vi "Register with Manager.vi"(8 "error in (no error)":errorcluster, 11 "HistorianCharting in":refnum<class "HistorianCharting.lvclass">) -> (0 "error out":errorcluster, 2 "Group Events":refnum<event-registration>, 3 "HistorianCharting out":refnum<class "HistorianCharting.lvclass">)   [LabVIEW 2020, in "VolatusGUIElements.lvlib" / "HistorianCharting.lvclass"]
uses:
  HistorianCharting.lvclass
  VolatusGUI/Historian Charting Manager/Plot Group Events.ctl
  VolatusGUI/Historian Charting Manager/Plot Group Changed Data.ctl
  VolatusGUI/Historian Charting Manager/Plot Group Config.ctl
  VolatusGUI/Historian Charting Manager/X-Axis Type.ctl
  VolatusGUI/Historian Charting Manager/Plot Config.ctl
  VolatusGUI/Historian Charting Manager/Scale.ctl
  VolatusGUI/Historian Charting Manager/Plot Group Removed Data.ctl
  VolatusGUI/Historian Charting Manager/New Plot Group Data.ctl
  VolatusGUI/Historian Charting Manager/Chart Select Group Data.ctl
  VolatusGUI/Historian Charting Manager/Chart Registration.ctl
  VolatusGUI/Historian Charting Manager/Select Plot Group Data.ctl
  VolatusGUI/Plot Group Events Value/Plot Group Events Value.lvclass
  HistorianCharting.lvclass/HistorianCharting.ctl
  VolatusGUI/Plot Group Events Value/Plot Group Events Value.lvclass/Plot Group Events Value.ctl
  VolatusGUI/Historian Charting Manager/Historian Charting Manager.lvclass
  Volatus/MessageQ/MessageQ.lvclass
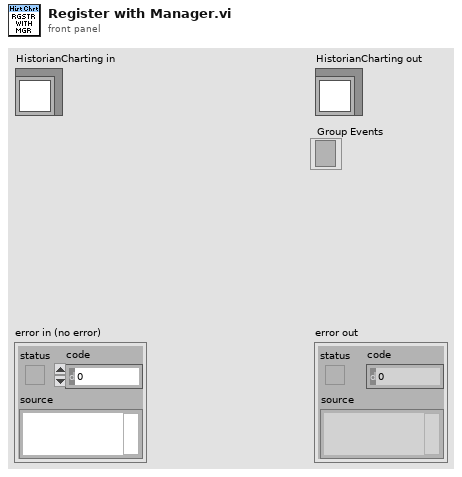
[diagram p1: front panel]
types:
  T1 = typedef "VolatusGUI.lvlib/Historian Charting Manager.lvclass/Chart Registration.ctl" = cluster{"Chart Num":i32, "Select Plot Group":refnum<user-event>}
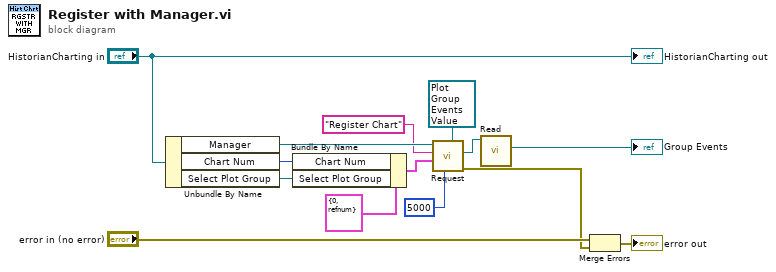
[diagram p0: block diagram]
diagram:
  n1 = Unbundle By Name("HistorianCharting in") -> ("Manager"=w9:refnum<class "MessageQ.lvclass">, "Chart Num"=w11:i32, "Select Plot Group"=w10:refnum<user-event>)
  n2 = Bundle By Name(cluster=T1 {"Chart Num"=0, "Select Plot Group"=refnum} ("Chart Registration"), "Chart Num"=w11, "Select Plot Group"=w10) -> (w7:T1)
  n3 = call "Request.vi"("Response Type (None)"=refnum<class "Plot Group Events Value.lvclass"> refnum ("VolatusGUI:Plot Group Events Value.lvclass"), "Timeout ms (1000)"=5000, "Data"=w7, "ID"="Register Chart", "MessageQ in"=w9) -> ("error out"=w5:errorcluster, "Response"=w2:refnum<class "Plot Group Events Value.lvclass">)  [unwired: 4 in, 1 out]
  n4 = call "Read.vi"("Plot Group Events Value in"=w2) -> ("Plot Group"=→"Group Events":refnum<event-registration>)  [unwired: 10 in]
  n5 = Merge Errors("error in (no error)", w5) -> (→"error out":errorcluster)
  "HistorianCharting out" <- "HistorianCharting in"
